vi "GeoData.vi"() -> ()   [LabVIEW 2017] (continued)
 County\tH1\n61476\t17131\tSeaton\tIL\tMercer County\tH1\n61472\t17131\tRio\tIL\tMercer County\tH1\n61262\t17131\tLynn center\tIL\tMercer County\tH1\n61259\t17131\tIllinois city\tIL\tMercer County\tH1\n61260\t17131\tJoy\tIL\tMercer County\tH1\n61264\t17131\tMilan\tIL\tMercer County\tH1\n61279\t17131\tReynolds\tIL\tMercer County\tH1\n61466\t17131\tNorth henderson\tIL\tMercer County\tH1\n61281\t17131\tSherrard\tIL\tMercer County\tH1\n61276\t17131\tPreemption\tIL\tMercer County\tH1\n61231\t17131\tAledo\tIL\tMercer County\tH1\n61273\t17131\tOrion\tIL\tMercer County\tH1\n61442\t17131\tKeithsburg\tIL\tMercer County\tH1\n62278\t17133\tRed bud\tIL\tMonroe County\tH1\n62236\t17133\tColumbia\tIL\tMonroe County\tH1\n62295\t17133\tValmeyer\tIL\tMonroe County\tH1\n62277\t17133\tPrairie du rocher\tIL\tMonroe County\tH1\n62264\t17133\tNew athens\tIL\tMonroe County\tH1\n62244\t17133\tFults\tIL\tMonroe County\tH1\n62248\t17133\tHecker\tIL\tMonroe County\tH1\n62298\t17133\tWaterloo\tIL\tMonroe County\tH1\n62256\t17133\tMaeystown\tIL\tMonroe County\tH1\n62240\t17133\tEast carondelet\tIL\tMonroe County\tH1\n62279\t17133\tRenault\tIL\tMonroe County\tH1\n62069\t17135\tMount olive\tIL\tMontgomery County\tH1\n62049\t17135\tHillsboro\tIL\tMontgomery County\tH1\n62560\t17135\tRaymond\tIL\tMontgomery County\tH1\n62019\t17135\tDonnellson\tIL\tMontgomery County\tH1\n62056\t17135\tLitchfield\tIL\tMontgomery County\tH1\n62032\t17135\tFillmore\tIL\tMontgomery County\tH1\n62076\t17135\tOhlman\tIL\tMontgomery County\tH1\n62533\t17135\tFarmersville\tIL\tMontgomery County\tH1\n62094\t17135\tWitt\tIL\tMontgomery County\tH1\n62083\t17135\tRosamond\tIL\tMontgomery County\tH1\n62262\t17135\tMulberry grove\tIL\tMontgomery County\tH1\n62553\t17135\tOconee\tIL\tMontgomery County\tH1\n62558\t17135\tPawnee\tIL\tMontgomery County\tH1\n62557\t17135\tPana\tIL\tMontgomery County\tH1\n62017\t17135\tCoffeen\tIL\tMontgomery County\tH1\n62086\t17135\tSorento\tIL\tMontgomery County\tH1\n62546\t17135\tMorrisonville\tIL\tMontgomery County\tH1\n62640\t17135\tGirard\tIL\tMontgomery County\tH1\n62075\t17135\tNokomis\tIL\tMontgomery County\tH1\n62091\t17135\tWalshville\tIL\tMontgomery County\tH1\n62077\t17135\tPanama\tIL\tMontgomery County\tH1\n62074\t17135\tNew douglas\tIL\tMontgomery County\tH1\n62080\t17135\tRamsey\tIL\tMontgomery County\tH1\n62089\t17135\tTaylor springs\tIL\tMontgomery County\tH1\n62051\t17135\tIrving\tIL\tMontgomery County\tH1\n62538\t17135\tHarvel\tIL\tMontgomery County\tH1\n62015\t17135\tButler\tIL\tMontgomery County\tH1\n62572\t17135\tWaggoner\tIL\tMontgomery County\tH1\n62690\t17135\tVirden\tIL\tMontgomery County\tH1\n62621\t17137\tBluffs\tIL\tMorgan County\tH1\n62692\t17137\tWaverly\tIL\tMorgan County\tH1\n62665\t17137\tMeredosia\tIL\tMorgan County\tH1\n62694\t17137\tWinchester\tIL\tMorgan County\tH1\n62667\t17137\tModesto\tIL\tMorgan County\tH1\n62650\t17137\tJacksonville\tIL\tMorgan County\tH1\n62677\t17137\tPleasant plains\tIL\tMorgan County\tH1\n62612\t17137\tAshland\tIL\tMorgan County\tH1\n62660\t17137\tLiterberry\tIL\tMorgan County\tH1\n62631\t17137\tConcord\tIL\tMorgan County\tH1\n62082\t17137\tRoodhouse\tIL\tMorgan County\tH1\n62695\t17137\tWoodson\tIL\tMorgan County\tH1\n62638\t17137\tFranklin\tIL\tMorgan County\tH1\n62670\t17137\tNew berlin\tIL\tMorgan County\tH1\n62668\t17137\tMurrayville\tIL\tMorgan County\tH1\n62601\t17137\tAlexander\tIL\tMorgan County\tH1\n62651\t17137\tJacksonville\tIL\tMorgan County\tH1\n62628\t17137\tChapin\tIL\tMorgan County\tH1\n62611\t17137\tArenzville\tIL\tMorgan County\tH1\n61937\t17139\tLovington\tIL\tMoultrie County\tH1\n61957\t17139\tWindsor\tIL\tMoultrie County\tH1\n61913\t17139\tAtwood\tIL\tMoultrie County\tH1\n61914\t17139\tBethany\tIL\tMoultrie County\tH1\n61925\t17139\tDalton city\tIL\tMoultrie County\tH1\n61911\t17139\tArthur\tIL\tMoultrie County\tH1\n61929\t17139\tHammond\tIL\tMoultrie County\tH1\n61951\t17139\tSullivan\tIL\tMoultrie County\tH1\n61928\t17139\tGays\tIL\tMoultrie County\tH1\n61047\t17141\tLeaf river\tIL\tOgle County\tH1\n61015\t17141\tChana\tIL\tOgle County\tH1\n61020\t17141\tDavis junction\tIL\tOgle County\tH1\n61039\t17141\tGerman valley\tIL\tOgle County\tH1\n60553\t17141\tSteward\tIL\tOgle County\tH1\n61006\t17141\tAshton\tIL\tOgle County\tH1\n61010\t17141\tByron\tIL\tOgle County\tH1\n61088\t17141\tWinnebago\tIL\tOgle County\tH1\n61068\t17141\tRochelle\tIL\tOgle County\tH1\n61054\t17141\tMount morris\tIL\tOgle County\tH1\n61051\t17141\tMilledgeville\tIL\tOgle County\tH1\n61064\t17141\tPolo\tIL\tOgle County\tH1\n61030\t17141\tForreston\tIL\tOgle County\tH1\n61091\t17141\tWoosung\tIL\tOgle County\tH1\n61052\t17141\tMonroe center\tIL\tOgle County\tH1\n61007\t17141\tBaileyville\tIL\tOgle County\tH1\n61031\t17141\tFranklin grove\tIL\tOgle County\tH1\n60113\t17141\tCreston\tIL\tOgle County\tH1\n61084\t17141\tStillman valley\tIL\tOgle County\tH1\n61109\t17141\tRockford\tIL\tOgle County\tH1\n61061\t17141\tOregon\tIL\tOgle County\tH1\n61078\t17141\tShannon\tIL\tOgle County\tH1\n60146\t17141\tKirkland\tIL\tOgle County\tH1\n61102\t17141\tRockford\tIL\tOgle County\tH1\n61021\t17141\tDixon\tIL\tOgle County\tH1\n60129\t17141\tEsmond\tIL\tOgle County\tH1\n61049\t17141\tLindenwood\tIL\tOgle County\tH1\n61043\t17141\tHolcomb\tIL\tOgle County\tH1\n61523\t17143\tChillicothe\tIL\tPeoria County\tH1\n61528\t17143\tEdwards\tIL\tPeoria County\tH1\n61529\t17143\tElmwood\tIL\tPeoria County\tH1\n61531\t17143\tFarmington\tIL\tPeoria County\tH1\n61605\t17143\tPeoria\tIL\tPeoria County\tH1\n61607\t17143\tPeoria\tIL\tPeoria County\tH1\n61601\t17143\tPeoria\tIL\tPeoria County\tH1\n61552\t17143\tMossville\tIL\tPeoria County\tH1\n61655\t17143\tPeoria\tIL\tPeoria County\tH1\n61639\t17143\tPeoria\tIL\tPeoria County\tH1\n61634\t17143\tPeoria\tIL\tPeoria County\tH1\n61520\t17143\tCanton\tIL\tPeoria County\tH1\n61565\t17143\tSparland\tIL\tPeoria County\tH1\n61651\t17143\tPeoria\tIL\tPeoria County\tH1\n61615\t17143\tPeoria\tIL\tPeoria County\tH1\n61604\t17143\tPeoria\tIL\tPeoria County\tH1\n61606\t17143\tPeoria\tIL\tPeoria County\tH1\n61562\t17143\tRome\tIL\tPeoria County\tH1\n61525\t17143\tDunlap\tIL\tPeoria County\tH1\n61526\t17143\tEdelstein\tIL\tPeoria County\tH1\n61536\t17143\tHanna city\tIL\tPeoria County\tH1\n61517\t17143\tBrimfield\tIL\tPeoria County\tH1\n61614\t17143\tPeoria\tIL\tPeoria County\tH1\n61451\t17143\tLaura\tIL\tPeoria County\tH1\n61539\t17143\tKingston mines\tIL\tPeoria County\tH1\n61629\t17143\tPeoria\tIL\tPeoria County\tH1\n61625\t17143\tPeoria\tIL\tPeoria County\tH1\n61638\t17143\tPeoria\tIL\tPeoria County\tH1\n61643\t17143\tPeoria\tIL\tPeoria County\tH1\n61479\t17143\tSpeer\tIL\tPeoria County\tH1\n61569\t17143\tTrivoli\tIL\tPeoria County\tH1\n61611\t17143\tEast peoria\tIL\tPeoria County\tH1\n61652\t17143\tPeoria\tIL\tPeoria County\tH1\n61654\t17143\tPeoria\tIL\tPeoria County\tH1\n61636\t17143\tPeoria\tIL\tPeoria County\tH1\n61616\t17143\tPeoria heights\tIL\tPeoria County\tH1\n61637\t17143\tPeoria\tIL\tPeoria County\tH1\n61656\t17143\tPeoria\tIL\tPeoria County\tH1\n61559\t17143\tPrinceville\tIL\tPeoria County\tH1\n61602\t17143\tPeoria\tIL\tPeoria County\tH1\n61612\t17143\tPeoria\tIL\tPeoria County\tH1\n61613\t17143\tPeoria\tIL\tPeoria County\tH1\n61533\t17143\tGlasford\tIL\tPeoria County\tH1\n61633\t17143\tPeoria\tIL\tPeoria County\tH1\n61603\t17143\tPeoria\tIL\tPeoria County\tH1\n61489\t17143\tWilliamsfield\tIL\tPeoria County\tH1\n61547\t17143\tMapleton\tIL\tPeoria County\tH1\n61653\t17143\tPeoria\tIL\tPeoria County\tH1\n61630\t17143\tPeoria\tIL\tPeoria County\tH1\n61641\t17143\tPeoria\tIL\tPeoria County\tH1\n62268\t17145\tOakdale\tIL\tPerry County\tH1\n62272\t17145\tPercy\tIL\tPerry County\tH1\n62907\t17145\tAva\tIL\tPerry County\tH1\n62916\t17145\tCampbell hill\tIL\tPerry County\tH1\n62997\t17145\tWillisville\tIL\tPerry County\tH1\n62274\t17145\tPinckneyville\tIL\tPerry County\tH1\n62263\t17145\tNashville\tIL\tPerry County\tH1\n62237\t17145\tCoulterville\tIL\tPerry County\tH1\n62831\t17145\tDu bois\tIL\tPerry County\tH1\n62883\t17145\tScheller\tIL\tPerry County\tH1\n62286\t17145\tSparta\tIL\tPerry County\tH1\n62832\t17145\tDu quoin\tIL\tPerry County\tH1\n62888\t17145\tTamaroa\tIL\tPerry County\tH1\n62238\t17145\tCutler\tIL\tPerry County\tH1\n61936\t17147\tLa place\tIL\tPiatt County\tH1\n61855\t17147\tMilmine\tIL\tPiatt County\tH1\n61813\t17147\tBement\tIL\tPiatt County\tH1\n61856\t17147\tMonticello\tIL\tPiatt County\tH1\n61839\t17147\tDe land\tIL\tPiatt County\tH1\n61937\t17147\tLovington\tIL\tPiatt County\tH1\n61884\t17147\tWhite heath\tIL\tPiatt County\tH1\n61851\t17147\tIvesdale\tIL\tPiatt County\tH1\n61882\t17147\tWeldon\tIL\tPiatt County\tH1\n61913\t17147\tAtwood\tIL\tPiatt County\tH1\n61842\t17147\tFarmer city\tIL\tPiatt County\tH1\n61853\t17147\tMahomet\tIL\tPiatt County\tH1\n61854\t17147\tMansfield\tIL\tPiatt County\tH1\n61929\t17147\tHammond\tIL\tPiatt County\tH1\n61818\t17147\tCerro gordo\tIL\tPiatt County\tH1\n61830\t17147\tCisco\tIL\tPiatt County\tH1\n61875\t17147\tSeymour\tIL\tPiatt County\tH1\n62314\t17149\tBaylis\tIL\tPike County\tH1\n62366\t17149\tPleasant hill\tIL\tPike County\tH1\n62370\t17149\tRockport\tIL\tPike County\tH1\n62345\t17149\tKinderhook\tIL\tPike County\tH1\n62363\t17149\tPittsfield\tIL\tPike County\tH1\n62355\t17149\tNebo\tIL\tPike County\tH1\n62343\t17149\tHull\tIL\tPike County\tH1\n62312\t17149\tBarry\tIL\tPike County\tH1\n62323\t17149\tChambersburg\tIL\tPike County\tH1\n62356\t17149\tNew canton\tIL\tPike County\tH1\n62340\t17149\tGriggsville\tIL\tPike County\tH1\n62357\t17149\tNew salem\tIL\tPike County\tH1\n62362\t17149\tPerry\tIL\tPike County\tH1\n62361\t17149\tPearl\tIL\tPike County\tH1\n62352\t17149\tMilton\tIL\tPike County\tH1\n62960\t17151\tMetropolis\tIL\tPope County\tH1\n62972\t17151\tOzark\tIL\tPope County\tH1\n62947\t17151\tHerod\tIL\tPope County\tH1\n62985\t17151\tSimpson\tIL\tPope County\tH1\n62987\t17151\tStonefort\tIL\tPope County\tH1\n62943\t17151\tGrantsburg\tIL\tPope County\tH1\n62938\t17151\tGolconda\tIL\tPope County\tH1\n62910\t17151\tBrookport\tIL\tPope County\tH1\n62928\t17151\tEddyville\tIL\tPope County\tH1\n62956\t17153\tKarnak\tIL\tPulaski County\tH1\n62963\t17153\tMound city\tIL\tPulaski County\tH1\n62996\t17153\tVilla ridge\tIL\tPulaski County\tH1\n62926\t17153\tDongola\tIL\tPulaski County\tH1\n62964\t17153\tMounds\tIL\tPulaski County\tH1\n62976\t17153\tPulaski\tIL\tPulaski County\tH1\n62973\t17153\tPerks\tIL\tPulaski County\tH1\n62970\t17153\tOlmsted\tIL\tPulaski County\tH1\n62992\t17153\tUllin\tIL\tPulaski County\tH1\n62923\t17153\tCypress\tIL\tPulaski County\tH1\n62941\t17153\tGrand chain\tIL\tPulaski County\tH1\n61560\t17155\tPutnam\tIL\tPutnam County\tH1\n61327\t17155\tHennepin\tIL\tPutnam County\tH1\n61363\t17155\tStandard\tIL\tPutnam County\tH1\n61336\t17155\tMagnolia\tIL\tPutnam County\tH1\n61335\t17155\tMc nabb\tIL\tPutnam County\tH1\n61334\t17155\tLostant\tIL\tPutnam County\tH1\n61326\t17155\tGranville\tIL\tPutnam County\tH1\n61340\t17155\tMark\tIL\tPutnam County\tH1\n62278\t17157\tRed bud\tIL\tRandolph County\tH1\n62272\t17157\tPercy\tIL\tRandolph County\tH1\n62277\t17157\tPrairie du rocher\tIL\tRandolph County\tH1\n62261\t17157\tModoc\tIL\tRandolph County\tH1\n62259\t17157\tMenard\tIL\tRandolph County\tH1\n62907\t17157\tAva\tIL\tRandolph County\tH1\n62916\t17157\tCampbell hill\tIL\tRandolph County\tH1\n62257\t17157\tMarissa\tIL\tRandolph County\tH1\n62297\t17157\tWalsh\tIL\tRandolph County\tH1\n62288\t17157\tSteeleville\tIL\tRandolph County\tH1\n62292\t17157\tTilden\tIL\tRandolph County\tH1\n62233\t17157\tChester\tIL\tRandolph County\tH1\n62237\t17157\tCoulterville\tIL\tRandolph County\tH1\n62242\t17157\tEvansville\tIL\tRandolph County\tH1\n62280\t17157\tRockwood\tIL\tRandolph County\tH1\n62217\t17157\tBaldwin\tIL\tRandolph County\tH1\n62286\t17157\tSparta\tIL\tRandolph County\tH1\n62241\t17157\tEllis grove\tIL\tRandolph County\tH1\n62238\t17157\tCutler\tIL\tRandolph County\tH1\n62448\t17159\tNewton\tIL\tRichland County\tH1\n62466\t17159\tSumner\tIL\tRichland County\tH1\n62450\t17159\tOlney\tIL\tRichland County\tH1\n62868\t17159\tNoble\tIL\tRichland County\tH1\n62425\t17159\tDundas\tIL\tRichland County\tH1\n62452\t17159\tParkersburg\tIL\tRichland County\tH1\n62421\t17159\tClaremont\tIL\tRichland County\tH1\n62476\t17159\tWest salem\tIL\tRichland County\tH1\n62419\t17159\tCalhoun\tIL\tRichland County\tH1\n61282\t17161\tSilvis\tIL\tRock Island County\tH1\n61266\t17161\tMoline\tIL\tRock Island County\tH1\n61237\t17161\tBuffalo prairie\tIL\tRock Island County\tH1\n61299\t17161\tRock island\tIL\tRock Island County\tH1\n61240\t17161\tCoal valley\tIL\tRock Island County\tH1\n61204\t17161\tRock island\tIL\tRock Island County\tH1\n61232\t17161\tAndalusia\tIL\tRock Island County\tH1\n61242\t17161\tCordova\tIL\tRock Island County\tH1\n61272\t17161\tNew boston\tIL\tRock Island County\tH1\n61278\t17161\tRapids city\tIL\tRock Island County\tH1\n61201\t17161\tRock island\tIL\tRock Island County\tH1\n61256\t17161\tHampton\tIL\tRock Island County\tH1\n61259\t17161\tIllinois city\tIL\tRock Island County\tH1\n61260\t17161\tJoy\tIL\tRock Island County\tH1\n61264\t17161\tMilan\tIL\tRock Island County\tH1\n61257\t17161\tHillsdale\tIL\tRock Island County\tH1\n61284\t17161\tTaylor ridge\tIL\tRock Island County\tH1\n61236\t17161\tBarstow\tIL\tRock Island County\tH1\n61265\t17161\tMoline\tIL\tRock Island County\tH1\n61279\t17161\tReynolds\tIL\tRock Island County\tH1\n61281\t17161\tSherrard\tIL\tRock Island County\tH1\n61239\t17161\tCarbon cliff\tIL\tRock Island County\tH1\n61275\t17161\tPort byron\tIL\tRock Island County\tH1\n61244\t17161\tEast moline\tIL\tRock Island County\tH1\n61273\t17161\tOrion\tIL\tRock Island County\tH1\n62223\t17163\tBelleville\tIL\tSt. Clair County\tH1\n62226\t17163\tBelleville\tIL\tSt. Clair County\tH1\n62236\t17163\tColumbia\tIL\tSt. Clair County\tH1\n62225\t17163\tScott air force base\tIL\tSt. Clair County\tH1\n62060\t17163\tMadison\tIL\tSt. Clair County\tH1\n62204\t17163\tEast saint louis\tIL\tSt. Clair County\tH1\n62232\t17163\tCaseyville\tIL\tSt. Clair County\tH1\n62264\t17163\tNew athens\tIL\tSt. Clair County\tH1\n62254\t17163\tLebanon\tIL\tSt. Clair County\tH1\n62071\t17163\tNational stock yards\tIL\tSt. Clair County\tH1\n62059\t17163\tLovejoy\tIL\tSt. Clair County\tH1\n62289\t17163\tSummerfield\tIL\tSt. Clair County\tH1\n62282\t17163\tSaint libory\tIL\tSt. Clair County\tH1\n62201\t17163\tEast saint louis\tIL\tSt. Clair County\tH1\n62239\t17163\tDupo\tIL\tSt. Clair County\tH1\n62260\t17163\tMillstadt\tIL\tSt. Clair County\tH1\n62298\t17163\tWaterloo\tIL\tSt. Clair County\tH1\n62269\t17163\tO fallon\tIL\tSt. Clair County\tH1\n62215\t17163\tAlbers\tIL\tSt. Clair County\tH1\n62257\t17163\tMarissa\tIL\tSt. Clair County\tH1\n62203\t17163\tEast saint louis\tIL\tSt. Clair County\tH1\n62234\t17163\tCollinsville\tIL\tSt. Clair County\tH1\n62207\t17163\tEast saint louis\tIL\tSt. Clair County\tH1\n62265\t17163\tNew baden\tIL\tSt. Clair County\tH1\n62222\t17163\tBelleville\tIL\tSt. Clair County\tH1\n62208\t17163\tFairview heights\tIL\tSt. Clair County\tH1\n62221\t17163\tBelleville\tIL\tSt. Clair County\tH1\n62240\t17163\tEast carondelet\tIL\tSt. Clair County\tH1\n62220\t17163\tBelleville\tIL\tSt. Clair County\tH1\n62243\t17163\tFreeburg\tIL\tSt. Clair County\tH1\n62205\t17163\tEast saint louis\tIL\tSt. Clair County\tH1\n62294\t17163\tTroy\tIL\tSt. Clair County\tH1\n62202\t17163\tEast saint louis\tIL\tSt. Clair County\tH1\n62285\t17163\tSmithton\tIL\tSt. Clair County\tH1\n62206\t17163\tEast saint louis\tIL\tSt. Clair County\tH1\n62258\t17163\tMascoutah\tIL\tSt. Clair County\tH1\n62255\t17163\tLenzburg\tIL\tSt. Clair County\tH1\n62293\t17163\tTrenton\tIL\tSt. Clair County\tH1\n62972\t17165\tOzark\tIL\tSaline County\tH1\n62917\t17165\tCarrier mills\tIL\tSaline County\tH1\n62965\t17165\tMuddy\tIL\tSaline County\tH1\n62947\t17165\tHerod\tIL\tSaline County\tH1\n62987\t17165\tStonefort\tIL\tSaline County\tH1\n62930\t17165\tEldorado\tIL\tSaline County\tH1\n62817\t17165\tBroughton\tIL\tSaline County\tH1\n62890\t17165\tThompsonville\tIL\tSaline County\tH1\n62935\t17165\tGalatia\tIL\tSaline County\tH1\n62934\t17165\tEquality\tIL\tSaline County\tH1\n62869\t17165\tNorris city\tIL\tSaline County\tH1\n62977\t17165\tRaleigh\tIL\tSaline County\tH1\n62946\t17165\tHarrisburg\tIL\tSaline County\tH1\n62545\t17167\tMechanicsburg\tIL\tSangamon County\tH1\n62615\t17167\tAuburn\tIL\tSangamon County\tH1\n62536\t17167\tGlenarm\tIL\tSangamon County\tH1\n62692\t17167\tWaverly\tIL\tSangamon County\tH1\n62769\t17167\tSpringfield\tIL\tSangamon County\tH1\n62765\t17167\tSpringfield\tIL\tSangamon County\tH1\n62548\t17167\tMount pulaski\tIL\tSangamon County\tH1\n62629\t17167\tChatham\tIL\tSangamon County\tH1\n62701\t17167\tSpringfield\tIL\tSangamon County\tH1\n62706\t17167\tSpringfield\tIL\tSangamon County\tH1\n62739\t17167\tSpringfield\tIL\tSangamon County\tH1\n62736\t17167\tSpringfield\tIL\tSangamon County\tH1\n62766\t17167\tSpringfield\tIL\tSangamon County\tH1\n62726\t17167\tSpringfield\tIL\tSangamon County\tH1\n62719\t17167\tSpringfield\tIL\tSangamon County\tH1\n62763\t17167\tSpringfield\tIL\tSangamon County\tH1\n62776\t17167\tSpringfield\tIL\tSangamon County\tH1\n62530\t17167\tDivernon\tIL\tSangamon County\tH1\n62625\t17167\tCantrall\tIL\tSangamon County\tH1\n62702\t17167\tSpringfield\tIL\tSangamon County\tH1\n62684\t17167\tSherman\tIL\tSangamon County\tH1\n62689\t17167\tThayer\tIL\tSangamon County\tH1\n62796\t17167\tSpringfield\tIL\tSangamon County\tH1\n62520\t17167\tDawson\tIL\tSangamon County\tH1\n62712\t17167\tSpringfield\tIL\tSangamon County\tH1\n62677\t17167\tPleasant plains\tIL\tSangamon County\tH1\n62612\t17167\tAshland\tIL\tSangamon County\tH1\n62708\t17167\tSpringfield\tIL\tSangamon County\tH1\n62791\t17167\tSpringfield\tIL\tSangamon County\tH1\n62722\t17167\tSpringfield\tIL\tSangamon County\tH1\n62715\t17167\tSpringfield\tIL\tSangamon County\tH1\n62662\t17167\tLowder\tIL\tSangamon County\tH1\n62558\t17167\tPawnee\tIL\tSangamon County\tH1\n62704\t17167\tSpringfield\tIL\tSangamon County\tH1\n62693\t17167\tWilliamsville\tIL\tSangamon County\tH1\n62705\t17167\tSpringfield\tIL\tSangamon County\tH1\n62539\t17167\tIlliopolis\tIL\tSangamon County\tH1\n62613\t17167\tAthens\tIL\tSangamon County\tH1\n62762\t17167\tSpringfield\tIL\tSangamon County\tH1\n62515\t17167\tBuffalo\tIL\tSangamon County\tH1\n62561\t17167\tRiverton\tIL\tSangamon County\tH1\n62703\t17167\tSpringfield\tIL\tSangamon County\tH1\n62661\t17167\tLoami\tIL\tSangamon County\tH1\n62764\t17167\tSpringfield\tIL\tSangamon County\tH1\n62756\t17167\tSpringfield\tIL\tSangamon County\tH1\n62781\t17167\tSpringfield\tIL\tSangamon County\tH1\n62711\t17167\tSpringfield\tIL\tSangamon County\tH1\n62670\t17167\tNew berlin\tIL\tSangamon County\tH1\n62707\t17167\tSpringfield\tIL\tSangamon County\tH1\n62723\t17167\tSpringfield\tIL\tSangamon County\tH1\n62767\t17167\tSpringfield\tIL\tSangamon County\tH1\n62563\t17167\tRochester\tIL\tSangamon County\tH1\n62690\t17167\tVirden\tIL\tSangamon County\tH1\n62757\t17167\tSpringfield\tIL\tSangamon County\tH1\n62716\t17167\tSpringfield\tIL\tSangamon County\tH1\n62624\t17169\tBrowning\tIL\tSchuyler County\tH1\n62681\t17169\tRushville\tIL\tSchuyler County\tH1\n61452\t17169\tLittleton\tIL\tSchuyler County\tH1\n62319\t17169\tCamden\tIL\tSchuyler County\tH1\n62346\t17169\tLa prairie\tIL\tSchuyler County\tH1\n62311\t17169\tAugusta\tIL\tSchuyler County\tH1\n62639\t17169\tFrederick\tIL\tSchuyler County\tH1\n62618\t17169\tBeardstown\tIL\tSchuyler County\tH1\n62344\t17169\tHuntsville\tIL\tSchuyler County\tH1\n61501\t17169\tAstoria\tIL\tSchuyler County\tH1\n62367\t17169\tPlymouth\tIL\tSchuyler County\tH1\n62621\t17171\tBluffs\tIL\tScott County\tH1\n62665\t17171\tMeredosia\tIL\tScott County\tH1\n62694\t17171\tWinchester\tIL\tScott County\tH1\n62610\t17171\tAlsey\tIL\tScott County\tH1\n62663\t17171\tManchester\tIL\tScott County\tH1\n62363\t17171\tPittsfield\tIL\tScott County\tH1\n62650\t17171\tJacksonville\tIL\tScott County\tH1\n62082\t17171\tRoodhouse\tIL\tScott County\tH1\n62668\t17171\tMurrayville\tIL\tScott County\tH1\n62628\t17171\tChapin\tIL\tScott County\tH1\n62465\t17173\tStrasburg\tIL\tShelby County\tH1\n62510\t17173\tAssumption\tIL\tShelby County\tH1\n62447\t17173\tNeoga\tIL\tShelby County\tH1\n62565\t17173\tShelbyville\tIL\tShelby County\tH1\n62463\t17173\tStewardson\tIL\tShelby County\tH1\n62571\t17173\tTower hill\tIL\tShelby County\tH1\n62414\t17173\tBeecher city\tIL\tShelby County\tH1\n62422\t17173\tCowden\tIL\tShelby County\tH1\n62534\t17173\tFindlay\tIL\tShelby County\tH1\n61957\t17173\tWindsor\tIL\tShelby County\tH1\n62431\t17173\tHerrick\tIL\tShelby County\tH1\n61914\t17173\tBethany\tIL\tShelby County\tH1\n62553\t17173\tOconee\tIL\tShelby County\tH1\n62557\t17173\tPana\tIL\tShelby County\tH1\n62444\t17173\tMode\tIL\tShelby County\tH1\n62544\t17173\tMacon\tIL\tShelby County\tH1\n62462\t17173\tSigel\tIL\tShelby County\tH1\n61951\t17173\tSullivan\tIL\tShelby County\tH1\n62550\t17173\tMoweaqua\tIL\tShelby County\tH1\n62438\t17173\tLakewood\tIL\tShelby County\tH1\n61928\t17173\tGays\tIL\tShelby County\tH1\n61449\t17175\tLa fayette\tIL\tStark County\tH1\n61483\t17175\tToulon\tIL\tStark County\tH1\n61426\t17175\tCastleton\tIL\tStark County\tH1\n61421\t17175\tBradford\tIL\tStark County\tH1\n61443\t17175\tKewanee\tIL\tStark County\tH1\n61479\t17175\tSpeer\tIL\tStark County\tH1\n61491\t17175\tWyoming\tIL\tStark County\tH1\n61559\t17175\tPrinceville\tIL\tStark County\tH1\n61434\t17175\tGalva\tIL\tStark County\tH1\n61047\t17177\tLeaf river\tIL\tStephenson County\tH1\n61039\t17177\tGerman valley\tIL\tStephenson County\tH1\n61087\t17177\tWarren\tIL\tStephenson County\tH1\n61089\t17177\tWinslow\tIL\tStephenson County\tH1\n61013\t17177\tCedarville\tIL\tStephenson County\tH1\n61062\t17177\tPearl city\tIL\tStephenson County\tH1\n61048\t17177\tLena\tIL\tStephenson County\tH1\n61044\t17177\tKent\tIL\tStephenson County\tH1\n61063\t17177\tPecatonica\tIL\tStephenson County\tH1\n61067\t17177\tRidott\tIL\tStephenson County\tH1\n61050\t17177\tMc connell\tIL\tStephenson County\tH1\n61007\t17177\tBaileyville\tIL\tStephenson County\tH1\n61070\t17177\tRock city\tIL\tStephenson County\tH1\n61018\t17177\tDakota\tIL\tStephenson County\tH1\n61027\t17177\tEleroy\tIL\tStephenson County\tH1\n61019\t17177\tDavis\tIL\tStephenson County\tH1\n61032\t17177\tFreeport\tIL\tStephenson County\tH1\n61078\t17177\tShannon\tIL\tStephenson County\tH1\n61060\t17177\tOrangeville\tIL\tStephenson County\tH1\n61546\t17179\tManito\tIL\tTazewell County\tH1\n61568\t17179\tTremont\tIL\tTazewell County\tH1\n61610\t17179\tCreve coeur\tIL\tTazewell County\tH1\n61548\t17179\tMetamora\tIL\tTazewell County\tH1\n61732\t17179\tDanvers\tIL\tTazewell County\tH1\n61759\t17179\tMinier\tIL\tTazewell County\tH1\n61550\t17179\tMorton\tIL\tTazewell County\tH1\n61535\t17179\tGroveland\tIL\tTazewell County\tH1\n61554\t17179\tPekin\tIL\tTazewell County\tH1\n61774\t17179\tStanford\tIL\tTazewell County\tH1\n61733\t17179\tDeer creek\tIL\tTazewell County\tH1\n61747\t17179\tHopedale\tIL\tTazewell County\tH1\n61635\t17179\tEast peoria\tIL\tTazewell County\tH1\n61734\t17179\tDelavan\tIL\tTazewell County\tH1\n62682\t17179\tSan jose\tIL\tTazewell County\tH1\n61534\t17179\tGreen valley\tIL\tTazewell County\tH1\n62635\t17179\tEmden\tIL\tTazewell County\tH1\n61558\t17179\tPekin\tIL\tTazewell County\tH1\n61611\t17179\tEast peoria\tIL\tTazewell County\tH1\n61755\t17179\tMackinaw\tIL\tTazewell County\tH1\n61555\t17179\tPekin\tIL\tTazewell County\tH1\n61742\t17179\tGoodfield\tIL\tTazewell County\tH1\n61564\t17179\tSouth pekin\tIL\tTazewell County\tH1\n61530\t17179\tEureka\tIL\tTazewell County\tH1\n61721\t17179\tArmington\tIL\tTazewell County\tH1\n61571\t17179\tWashington\tIL\tTazewell County\tH1\n62952\t17181\tJonesboro\tIL\tUnion County\tH1\n62957\t17181\tMc clure\tIL\tUnion County\tH1\n62905\t17181\tAlto pass\tIL\tUnion County\tH1\n62958\t17181\tMakanda\tIL\tUnion County\tH1\n62912\t17181\tBuncombe\tIL\tUnion County\tH1\n62961\t17181\tMillcreek\tIL\tUnion County\tH1\n62926\t17181\tDongola\tIL\tUnion County\tH1\n62939\t17181\tGoreville\tIL\tUnion County\tH1\n62998\t17181\tWolf lake\tIL\tUnion County\tH1\n62906\t17181\tAnna\tIL\tUnion County\tH1\n62920\t17181\tCobden\tIL\tUnion County\tH1\n62902\t17181\tCarbondale\tIL\tUnion County\tH1\n62988\t17181\tTamms\tIL\tUnion County\tH1\n62923\t17181\tCypress\tIL\tUnion County\tH1\n61841\t17183\tFairmount\tIL\tVermilion County\tH1\n61844\t17183\tFithian\tIL\tVermilion County\tH1\n61876\t17183\tSidell\tIL\tVermilion County\tH1\n60932\t17183\tEast lynn\tIL\tVermilion County\tH1\n61859\t17183\tOgden\tIL\tVermilion County\tH1\n61858\t17183\tOakwood\tIL\tVermilion County\tH1\n61862\t17183\tPenfield\tIL\tVermilion County\tH1\n61831\t17183\tCollison\tIL\tVermilion County\tH1\n61834\t17183\tDanville\tIL\tVermilion County\tH1\n61846\t17183\tGeorgetown\tIL\tVermilion County\tH1\n61833\t17183\tTilton\tIL\tVermilion County\tH1\n61850\t17183\tIndianola\tIL\tVermilion County\tH1\n60960\t17183\tRankin\tIL\tVermilion County\tH1\n61812\t17183\tArmstrong\tIL\tVermilion County\tH1\n61814\t17183\tBismarck\tIL\tVermilion County\tH1\n61849\t17183\tHomer\tIL\tVermilion County\tH1\n60963\t17183\tRossville\tIL\tVermilion County\tH1\n61832\t17183\tDanville\tIL\tVermilion County\tH1\n61810\t17183\tAllerton\tIL\tVermilion County\tH1\n61857\t17183\tMuncie\tIL\tVermilion County\tH1\n60942\t17183\tHoopeston\tIL\tVermilion County\tH1\n61817\t17183\tCatlin\tIL\tVermilion County\tH1\n61811\t17183\tAlvin\tIL\tVermilion County\tH1\n61883\t17183\tWestville\tIL\tVermilion County\tH1\n61865\t17183\tPotomac\tIL\tVermilion County\tH1\n61848\t17183\tHenning\tIL\tVermilion County\tH1\n61870\t17183\tRidge farm\tIL\tVermilion County\tH1\n62410\t17185\tAllendale\tIL\tWabash County\tH1\n62852\t17185\tKeensburg\tIL\tWabash County\tH1\n62811\t17185\tBellmont\tIL\tWabash County\tH1\n62818\t17185\tBrowns\tIL\tWabash County\tH1\n62476\t17185\tWest salem\tIL\tWabash County\tH1\n62863\t17185\tMount carmel\tIL\tWabash County\tH1\n62460\t17185\tSaint francisville\tIL\tWabash County\tH1\n61412\t17187\tAlexis\tIL\tWarren County\tH1\n61415\t17187\tAvon\tIL\tWarren County\tH1\n61418\t17187\tBiggsville\tIL\tWarren County\tH1\n61417\t17187\tBerwick\tIL\tWarren County\tH1\n61475\t17187\tSciota\tIL\tWarren County\tH1\n61410\t17187\tAbingdon\tIL\tWarren County\tH1\n61423\t17187\tCameron\tIL\tWarren County\tH1\n61401\t17187\tGalesburg\tIL\tWarren County\tH1\n61476\t17187\tSeaton\tIL\tWarren County\tH1\n61473\t17187\tRoseville\tIL\tWarren County\tH1\n61435\t17187\tGerlaw\tIL\tWarren County\tH1\n61462\t17187\tMonmouth\tIL\tWarren County\tH1\n61438\t17187\tGood hope\tIL\tWarren County\tH1\n61478\t17187\tSmithshire\tIL\tWarren County\tH1\n61466\t17187\tNorth henderson\tIL\tWarren County\tH1\n61453\t17187\tLittle york\tIL\tWarren County\tH1\n61447\t17187\tKirkwood\tIL\tWarren County\tH1\n61474\t17187\tSaint augustine\tIL\tWarren County\tH1\n62268\t17189\tOakdale\tIL\tWashington County\tH1\n62271\t17189\tOkawville\tIL\tWashington County\tH1\n62876\t17189\tRadom\tIL\tWashington County\tH1\n62848\t17189\tIrvington\tIL\tWashington County\tH1\n62801\t17189\tCentralia\tIL\tWashington County\tH1\n62803\t17189\tHoyleton\tIL\tWashington County\tH1\n62808\t17189\tAshley\tIL\tWashington County\tH1\n62257\t17189\tMarissa\tIL\tWashington County\tH1\n62214\t17189\tAddieville\tIL\tWashington County\tH1\n62263\t17189\tNashville\tIL\tWashington County\tH1\n62237\t17189\tCoulterville\tIL\tWashington County\tH1\n62831\t17189\tDu bois\tIL\tWashington County\tH1\n62877\t17189\tRichview\tIL\tWashington County\tH1\n62255\t17189\tLenzburg\tIL\tWashington County\tH1\n62837\t17191\tFairfield\tIL\tWayne County\tH1\n62886\t17191\tSims\tIL\tWayne County\tH1\n62823\t17191\tCisne\tIL\tWayne County\tH1\n62878\t17191\tRinard\tIL\tWayne County\tH1\n62828\t17191\tDahlgren\tIL\tWayne County\tH1\n62899\t17191\tXenia\tIL\tWayne County\tH1\n62446\t17191\tMount erie\tIL\tWayne County\tH1\n62820\t17191\tBurnt praire\tIL\tWayne County\tH1\n62851\t17191\tKeenes\tIL\tWayne County\tH1\n62833\t17191\tEllery\tIL\tWayne County\tH1\n62809\t17191\tBarnhill\tIL\tWayne County\tH1\n62839\t17191\tFlora\tIL\tWayne County\tH1\n62868\t17191\tNoble\tIL\tWayne County\tH1\n62895\t17191\tWayne city\tIL\tWayne County\tH1\n62814\t17191\tBluford\tIL\tWayne County\tH1\n62824\t17191\tClay city\tIL\tWayne County\tH1\n62842\t17191\tGeff\tIL\tWayne County\tH1\n62850\t17191\tJohnsonville\tIL\tWayne County\tH1\n62843\t17191\tGolden gate\tIL\tWayne County\tH1\n62821\t17193\tCarmi\tIL\tWhite County\tH1\n62861\t17193\tMaunie\tIL\tWhite County\tH1\n62834\t17193\tEmma\tIL\tWhite County\tH1\n62867\t17193\tNew haven\tIL\tWhite County\tH1\n62820\t17193\tBurnt praire\tIL\tWhite County\tH1\n62844\t17193\tGrayville\tIL\tWhite County\tH1\n62818\t17193\tBrowns\tIL\tWhite County\tH1\n62835\t17193\tEnfield\tIL\tWhite County\tH1\n62827\t17193\tCrossville\tIL\tWhite County\tH1\n62887\t17193\tSpringerton\tIL\tWhite County\tH1\n62869\t17193\tNorris city\tIL\tWhite County\tH1\n62862\t17193\tMill shoals\tIL\tWhite County\tH1\n61254\t17195\tGeneseo\tIL\tWhiteside County\tH1\n61261\t17195\tLyndon\tIL\tWhiteside County\tH1\n61042\t17195\tHarmon\tIL\tWhiteside County\tH1\n61283\t17195\tTampico\tIL\tWhiteside County\tH1\n61051\t17195\tMilledgeville\tIL\tWhiteside County\tH1\n61064\t17195\tPolo\tIL\tWhiteside County\tH1\n61243\t17195\tDeer grove\tIL\tWhiteside County\tH1\n61252\t17195\tFulton\tIL\tWhiteside County\tH1\n61081\t17195\tSterling\tIL\tWhiteside County\tH1\n61376\t17195\tWalnut\tIL\tWhiteside County\tH1\n61037\t17195\tGalt\tIL\tWhiteside County\tH1\n61270\t17195\tMorrison\tIL\tWhiteside County\tH1\n61277\t17195\tProphetstown\tIL\tWhiteside County\tH1\n61250\t17195\tErie\tIL\tWhiteside County\tH1\n61071\t17195\tRock falls\tIL\tWhiteside County\tH1\n61014\t17195\tChadwick\tIL\tWhiteside County\tH1\n61230\t17195\tAlbany\tIL\tWhiteside County\tH1\n61251\t17195\tFenton\tIL\tWhiteside County\tH1\n60403\t17197\tCrest hill\tIL\tWill County\tH1\n60417\t17197\tCrete\tIL\tWill County\tH1\n60481\t17197\tWilmington\tIL\tWill County\tH1\n60517\t17197\tWoodridge\tIL\tWill County\tH1\n60439\t17197\tLemont\tIL\tWill County\tH1\n60423\t17197\tFrankfort\tIL\tWill County\tH1\n60564\t17197\tNaperville\tIL\tWill County\tH1\n60544\t17197\tPlainfield\tIL\tWill County\tH1\n60585\t17197\tPlainfield\tIL\tWill County\tH1\n60935\t17197\tEssex\tIL\tWill County\tH1\n60411\t17197\tChicago heights\tIL\tWill County\tH1\n60401\t17197\tBeecher\tIL\tWill County\tH1\n60408\t17197\tBraidwood\tIL\tWill County\tH1\n60431\t17197\tJoliet\tIL\tWill County\tH1\n60433\t17197\tJoliet\tIL\tWill County\tH1\n60490\t17197\tBolingbrook\tIL\tWill County\tH1\n60503\t17197\tAurora\tIL\tWill County\tH1\n60407\t17197\tBraceville\tIL\tWill County\tH1\n60410\t17197\tChannahon\tIL\tWill County\tH1\n60435\t17197\tJoliet\tIL\tWill County\tH1\n60441\t17197\tLockport\tIL\tWill County\tH1\n60451\t17197\tNew lenox\tIL\tWill County\tH1\n60446\t17197\tRomeoville\tIL\tWill County\tH1\n60471\t17197\tRichton park\tIL\tWill County\tH1\n60567\t17197\tNaperville\tIL\tWill County\tH1\n60543\t17197\tOswego\tIL\tWill County\tH1\n60565\t17197\tNaperville\tIL\tWill County\tH1\n60950\t17197\tManteno\tIL\tWill County\tH1\n60447\t17197\tMinooka\tIL\tWill County\tH1\n60440\t17197\tBolingbrook\tIL\tWill County\tH1\n60448\t17197\tMokena\tIL\tWill County\tH1\n60487\t17197\tTinley park\tIL\tWill County\tH1\n60466\t17197\tPark forest\tIL\tWill County\tH1\n60416\t17197\tCoal city\tIL\tWill County\tH1\n60432\t17197\tJoliet\tIL\tWill County\tH1\n60586\t17197\tPlainfield\tIL\tWill County\tH1\n60434\t17197\tJoliet\tIL\tWill County\tH1\n60404\t17197\tShorewood\tIL\tWill County\tH1\n60449\t17197\tMonee\tIL\tWill County\tH1\n60421\t17197\tElwood\tIL\tWill County\tH1\n60477\t17197\tTinley park\tIL\tWill County\tH1\n60468\t17197\tPeotone\tIL\tWill County\tH1\n60484\t17197\tUniversity park\tIL\tWill County\tH1\n60940\t17197\tGrant park\tIL\tWill County\tH1\n60442\t17197\tManhattan\tIL\tWill County\tH1\n60436\t17197\tJoliet\tIL\tWill County\tH1\n60491\t17197\tHomer glen\tIL\tWill County\tH1\n60467\t17197\tOrland park\tIL\tWill County\tH1\n60475\t17197\tSteger\tIL\tWill County\tH1\n62918\t17199\tCarterville\tIL\tWilliamson County\tH1\n62972\t17199\tOzark\tIL\tWilliamson County\tH1\n62917\t17199\tCarrier mills\tIL\tWilliamson County\tH1\n62921\t17199\tColp\tIL\tWilliamson County\tH1\n62974\t17199\tPittsburg\tIL\tWilliamson County\tH1\n62987\t17199\tStonefort\tIL\tWilliamson County\tH1\n62933\t17199\tEnergy\tIL\tWilliamson County\tH1\n62841\t17199\tFreeman spur\tIL\tWilliamson County\tH1\n62896\t17199\tWest frankfort\tIL\tWilliamson County\tH1\n62948\t17199\tHerrin\tIL\tWilliamson County\tH1\n62958\t17199\tMakanda\tIL\tWilliamson County\tH1\n62924\t17199\tDe soto\tIL\tWilliamson County\tH1\n62939\t17199\tGoreville\tIL\tWilliamson County\tH1\n62922\t17199\tCreal springs\tIL\tWilliamson County\tH1\n62915\t17199\tCambria\tIL\tWilliamson County\tH1\n62949\t17199\tHurst\tIL\tWilliamson County\tH1\n62890\t17199\tThompsonville\tIL\tWilliamson County\tH1\n62951\t17199\tJohnston city\tIL\tWilliamson County\tH1\n62901\t17199\tCarbondale\tIL\tWilliamson County\tH1\n62959\t17199\tMarion\tIL\tWilliamson County\tH1\n62902\t17199\tCarbondale\tIL\tWilliamson County\tH1\n61047\t17201\tLeaf river\tIL\tWinnebago County\tH1\n61114\t17201\tRockford\tIL\tWinnebago County\tH1\n61020\t17201\tDavis junction\tIL\tWinnebago County\tH1\n61011\t17201\tCaledonia\tIL\tWinnebago County\tH1\n61039\t17201\tGerman valley\tIL\tWinnebago County\tH1\n61110\t17201\tRockford\tIL\tWinnebago County\tH1\n61104\t17201\tRockford\tIL\tWinnebago County\tH1\n61115\t17201\tMachesney park\tIL\tWinnebago County\tH1\n61132\t17201\tLoves park\tIL\tWinnebago County\tH1\n61079\t17201\tShirland\tIL\tWinnebago County\tH1\n61008\t17201\tBelvidere\tIL\tWinnebago County\tH1\n61101\t17201\tRockford\tIL\tWinnebago County\tH1\n61073\t17201\tRoscoe\tIL\tWinnebago County\tH1\n61088\t17201\tWinnebago\tIL\tWinnebago County\tH1\n61080\t17201\tSouth beloit\tIL\tWinnebago County\tH1\n61063\t17201\tPecatonica\tIL\tWinnebago County\tH1\n61024\t17201\tDurand\tIL\tWinnebago County\tH1\n61072\t17201\tRockton\tIL\tWinnebago County\tH1\n61112\t17201\tRockford\tIL\tWinnebago County\tH1\n61052\t17201\tMonroe center\tIL\tWinnebago County\tH1\n61111\t17201\tLoves park\tIL\tWinnebago County\tH1\n61131\t17201\tLoves park\tIL\tWinnebago County\tH1\n61077\t17201\tSeward\tIL\tWinnebago County\tH1\n61130\t17201\tLoves park\tIL\tWinnebago County\tH1\n61084\t17201\tStillman valley\tIL\tWinnebago County\tH1\n61107\t17201\tRockford\tIL\tWinnebago County\tH1\n61109\t17201\tRockford\tIL\tWinnebago County\tH1\n61125\t17201\tRockford\tIL\tWinnebago County\tH1\n61108\t17201\tRockford\tIL\tWinnebago County\tH1\n61019\t17201\tDavis\tIL\tWinnebago County\tH1\n61105\t17201\tRockford\tIL\tWinnebago County\tH1\n60146\t17201\tKirkland\tIL\tWinnebago County\tH1\n61102\t17201\tRockford\tIL\tWinnebago County\tH1\n61103\t17201\tRockford\tIL\tWinnebago County\tH1\n61126\t17201\tRockford\tIL\tWinnebago County\tH1\n61016\t17201\tCherry valley\tIL\tWinnebago County\tH1\n61744\t17203\tGridley\tIL\tWoodford County\tH1\n61771\t17203\tSecor\tIL\tWoodford County\tH1\n61548\t17203\tMetamora\tIL\tWoodford County\tH1\n61732\t17203\tDanvers\tIL\tWoodford County\tH1\n61570\t17203\tWashburn\tIL\tWoodford County\tH1\n61733\t17203\tDeer creek\tIL\tWoodford County\tH1\n61611\t17203\tEast peoria\tIL\tWoodford County\tH1\n61516\t17203\tBenson\tIL\tWoodford County\tH1\n61725\t17203\tCarlock\tIL\tWoodford County\tH1\n61748\t17203\tHudson\tIL\tWoodford County\tH1\n61742\t17203\tGoodfield\tIL\tWoodford County\tH1\n61729\t17203\tCongerville\tIL\tWoodford County\tH1\n61530\t17203\tEureka\tIL\tWoodford County\tH1\n61738\t17203\tEl paso\tIL\tWoodford County\tH1\n61321\t17203\tDana\tIL\tWoodford County\tH1\n61545\t17203\tLowpoint\tIL\tWoodford County\tH1\n61571\t17203\tWashington\tIL\tWoodford County\tH1\n61561\t17203\tRoanoke\tIL\tWoodford County\tH1\n61760\t17203\tMinonk\tIL\tWoodford County\tH1\n46780\t18001\tPleasant mills\tIN\tAdams County\tH1\n46773\t18001\tMonroeville\tIN\tAdams County\tH1\n46714\t18001\tBluffton\tIN\tAdams County\tH1\n46777\t18001\tOssian\tIN\tAdams County\tH1\n47326\t18001\tBryant\tIN\tAdams County\tH1\n46740\t18001\tGeneva\tIN\tAdams County\tH1\n46772\t18001\tMonroe\tIN\tAdams County\tH1\n46769\t18001\tLinn grove\tIN\tAdams County\tH1\n46782\t18001\tPreble\tIN\tAdams County\tH1\n46711\t18001\tBerne\tIN\tAdams County\tH1\n46745\t18001\tHoagland\tIN\tAdams County\tH1\n46731\t18001\tCraigville\tIN\tAdams County\tH1\n46733\t18001\tDecatur\tIN\tAdams County\tH1\n46725\t18003\tColumbia city\tIN\tAllen County\tH1\n46808\t18003\tFort wayne\tIN\tAllen County\tH1\n46798\t18003\tYoder\tIN\tAllen County\tH1\n46898\t18003\tFort wayne\tIN\tAllen County\tH1\n46819\t18003\tFort wayne\tIN\tAllen County\tH1\n46850\t18003\tFort wayne\tIN\tAllen County\tH1\n46867\t18003\tFort wayne\tIN\tAllen County\tH1\n46868\t18003\tFort wayne\tIN\tAllen County\tH1\n46860\t18003\tFort wayne\tIN\tAllen County\tH1\n46859\t18003\tFort wayne\tIN\tAllen County\tH1\n46773\t18003\tMonroeville\tIN\tAllen County\tH1\n46809\t18003\tFort wayne\tIN\tAllen County\tH1\n46777\t18003\tOssian\tIN\tAllen County\tH1\n46783\t18003\tRoanoke\tIN\tAllen County\tH1\n46899\t18003\tFort wayne\tIN\tAllen County\tH1\n46863\t18003\tFort wayne\tIN\tAllen County\tH1\n46853\t18003\tFort wayne\tIN\tAllen County\tH1\n46748\t18003\tHuntertown\tIN\tAllen County\tH1\n46804\t18003\tFort wayne\tIN\tAllen County\tH1\n46855\t18003\tFort wayne\tIN\tAllen County\tH1\n46743\t18003\tHarlan\tIN\tAllen County\tH1\n46806\t18003\tFort wayne\tIN\tAllen County\tH1\n46799\t18003\tZanesville\tIN\tAllen County\tH1\n46869\t18003\tFort wayne\tIN\tAllen County\tH1\n46895\t18003\tFort wayne\tIN\tAllen County\tH1\n46865\t18003\tFort wayne\tIN\tAllen County\tH1\n46797\t18003\tWoodburn\tIN\tAllen County\tH1\n46774\t18003\tNew haven\tIN\tAllen County\tH1\n46856\t18003\tFort wayne\tIN\tAllen County\tH1\n46861\t18003\tFort wayne\tIN\tAllen County\tH1\n46885\t18003\tFort wayne\tIN\tAllen County\tH1\n46805\t18003\tFort wayne\tIN\tAllen County\tH1\n46745\t18003\tHoagland\tIN\tAllen County\tH1\n46814\t18003\tFort wayne\tIN\tAllen County\tH1\n46803\t18003\tFort wayne\tIN\tAllen County\tH1\n46845\t18003\tFort wayne\tIN\tAllen County\tH1\n46862\t18003\tFort wayne\tIN\tAllen County\tH1\n46704\t18003\tArcola\tIN\tAllen County\tH1\n46852\t18003\tFort wayne\tIN\tAllen County\tH1\n46864\t18003\tFort wayne\tIN\tAllen County\tH1\n46857\t18003\tFort wayne\tIN\tAllen County\tH1\n46765\t18003\tLeo\tIN\tAllen County\tH1\n46706\t18003\tAuburn\tIN\tAllen County\tH1\n46825\t18003\tFort wayne\tIN\tAllen County\tH1\n46835\t18003\tFort wayne\tIN\tAllen County\tH1\n46816\t18003\tFort wayne\tIN\tAllen County\tH1\n46866\t18003\tFort wayne\tIN\tAllen County\tH1\n46851\t18003\tFort wayne\tIN\tAllen County\tH1\n46858\t18003\tFort wayne\tIN\tAllen County\tH1\n46723\t18003\tChurubusco\tIN\tAllen County\tH1\n46733\t18003\tDecatur\tIN\tAllen County\tH1\n46741\t18003\tGrabill\tIN\tAllen County\tH1\n46807\t18003\tFort wayne\tIN\tAllen County\tH1\n46788\t18003\tSpencerville\tIN\tAllen County\tH1\n46802\t18003\tFort wayne\tIN\tAllen County\tH1\n46818\t18003\tFort wayne\tIN\tAllen County\tH1\n46815\t18003\tFort wayne\tIN\tAllen County\tH1\n46854\t18003\tFort wayne\tIN\tAllen County\tH1\n47274\t18005\tSeymour\tIN\tBartholomew County\tH1\n47448\t18005\tNashville\tIN\tBartholomew County\tH1\n47202\t18005\tColumbus\tIN\tBartholomew County\tH1\n47273\t18005\tScipio\tIN\tBartholomew County\tH1\n47247\t18005\tJonesville\tIN\tBartholomew County\tH1\n47232\t18005\tElizabethtown\tIN\tBartholomew County\tH1\n47283\t18005\tWestport\tIN\tBartholomew County\tH1\n47203\t18005\tColumbus\tIN\tBartholomew County\tH1\n47236\t18005\tGrammer\tIN\tBartholomew County\tH1\n47201\t18005\tColumbus\tIN\tBartholomew County\tH1\n47280\t18005\tTaylorsville\tIN\tBartholomew County\tH1\n46124\t18005\tEdinburgh\tIN\tBartholomew County\tH1\n47246\t18005\t
